vi "PositionToCVT.vi"(8 "error in (no error)":errorcluster, 9 "Position Array":dbl[](array[numeric]), 11 "Connected Axes":string[](array[string])) -> (0 "error out":errorcluster)   [LabVIEW 2020]
uses:
  shared/CompressAndUpdate(Poly)/CompressAndUpdate(Numeric).vi
panel:
  out "Variable to update":string
  out "Value":dbl
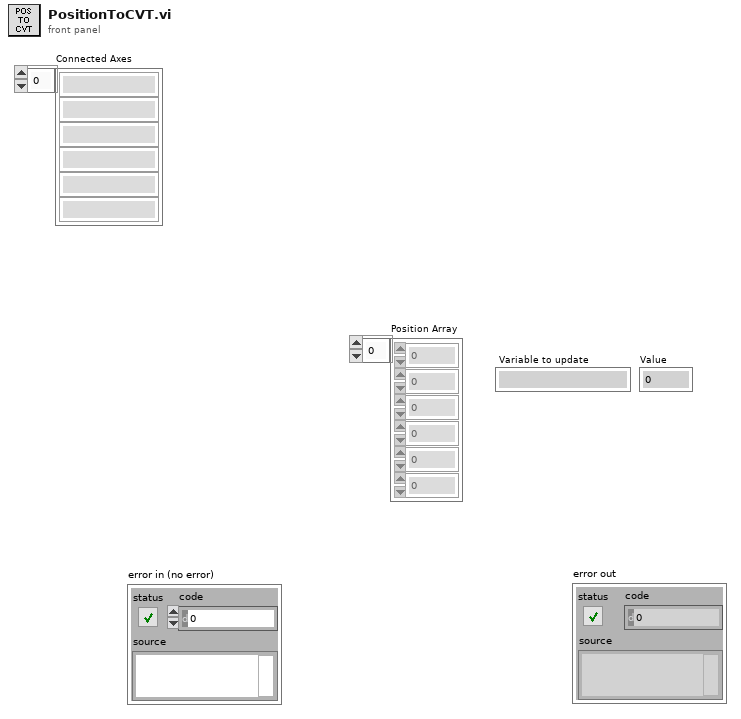
[diagram p1: front panel]
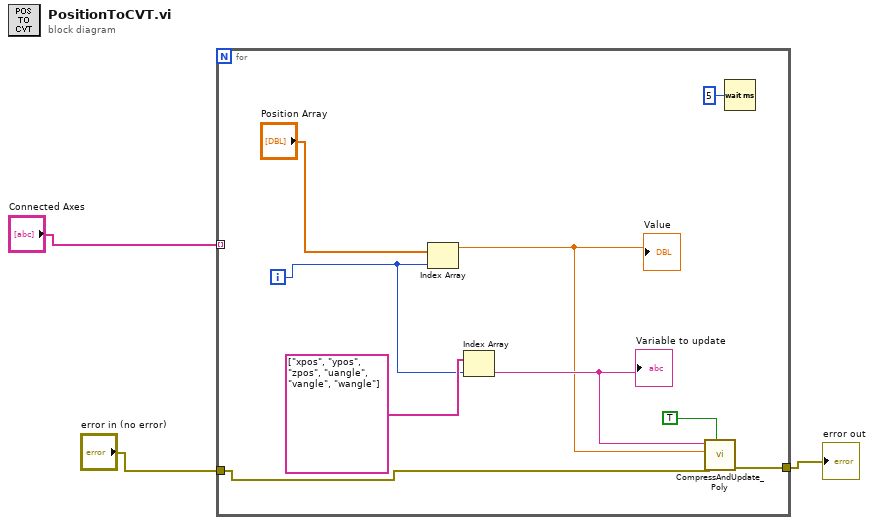
[diagram p0: block diagram]
diagram:
  n1 = for {
    tunnel: "Connected Axes" -> [_] mode=indexing
    tunnel: [w6] -> w1
    tunnel: "error in (no error)" -> [w5]
    i -> [w10]
    n2 = Index Array(array="Position Array", index=w10) -> (element=w8:dbl)
    "Value" <- w8
    n3 = Index Array(array=string[] ["xpos", "ypos", "zpos", "uangle", "vangle", "wangle"], index=w10) -> (element=w9:string)
    "Variable to update" <- w9
    n4 = call-poly "CompressAndUpdate_Poly.vi"("force CVT update (false)"=TRUE, "error in"=w5, "Numeric"=w8, "command or variable name"=w9) -> ("error out"=w6:errorcluster)  [unwired: 7 in]
    n5 = Wait (ms)(milliseconds to wait=u32 5) -> ()  [unwired: 1 out]
  }
  "error out" <- w1
